vi "setM1M3SAL.vi"(10 "M1M3SAL":refnum<class "M1M3SAL.lvclass">, 11 "Publisher in":refnum<class "Publisher.lvclass">) -> (3 "Publisher out":refnum<class "Publisher.lvclass">)   [LabVIEW 2016, in "Publisher.lvclass"]
uses:
  Publisher.lvclass
  Communicator/M1M3SAL/M1M3SAL.lvclass
  Publisher.lvclass/Publisher.ctl
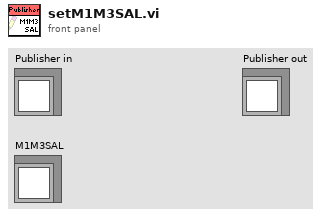
[diagram p1: front panel]
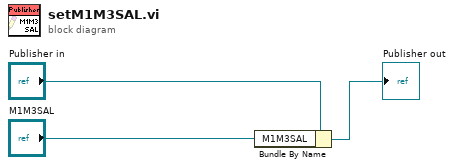
[diagram p0: block diagram]
diagram:
  n1 = Bundle By Name(cluster="Publisher in", "M1M3SAL"="M1M3SAL") -> (→"Publisher out":refnum<class "Publisher.lvclass">)
